vi "Handle Last Ack Core.vi"(4 "error in (no error)":errorcluster, 6 "Last Ack":refnum<class "Last Ack.lvclass">, 7 "Controller in":refnum<class "Controller.lvclass">) -> (0 "error out":errorcluster, 3 "Controller out":refnum<class "Controller.lvclass">)   [LabVIEW 2016, in "Controller Actor.lvlib" / "Controller.lvclass"]
doc: "(<B>Filename</B>: Actor Framework.lvlib:Actor.lvclass:Handle Last Ack Core.vi)\n\nDefines how the caller actor responds to the Last Ack message from a nested actor. The Last Ack message is the final message a nested actor sends to its caller before it shuts down. The message contains information about the final state of the nested actor.\n\nBy default, this method does nothing except return any error the nested actor sent. A descendant class may override this method to define behavior."
uses:
  <userlib>/Common Components/Controller/Controller.lvclass
  <vilib>/ActorFramework/LastAck/Last Ack.lvclass
  <vilib>/ActorFramework/LastAck/Last Ack.lvclass/Last Ack.ctl
  <userlib>/Configuration Dialog Actor/Configuration.lvclass
  <userlib>/Configuration Dialog Actor/Configuration.lvclass/Configuration.ctl
  <userlib>/Common Components/Controller/Controller.lvclass/Controller.ctl
  <vilib>/ActorFramework/Message Enqueuer/Message Enqueuer.lvclass/Message Enqueuer.ctl
  <userlib>/Common Components/Function Actor/Function.lvclass
  <userlib>/Common Components/Function Actor/Function.lvclass/Function.ctl
  <vilib>/ActorFramework/Message Enqueuer/Enqueue.vi
  <userlib>/Common Components/User Interface/Messages/Enable UI Msg/Enable UI Msg.lvclass
  C:/Program Files (x86)/National Instruments/LabVIEW 2016/vi.lib/ActorFramework/Message/Message.lvclass
  <vilib>/ActorFramework/Message Priority Queue/Priority Enqueue.vi
  <vilib>/ActorFramework/Actor/Actor.lvclass
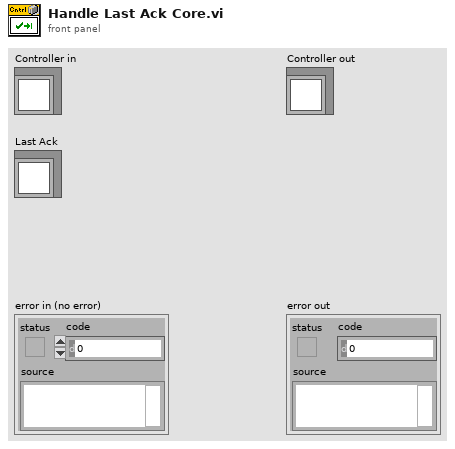
[diagram p1: front panel]
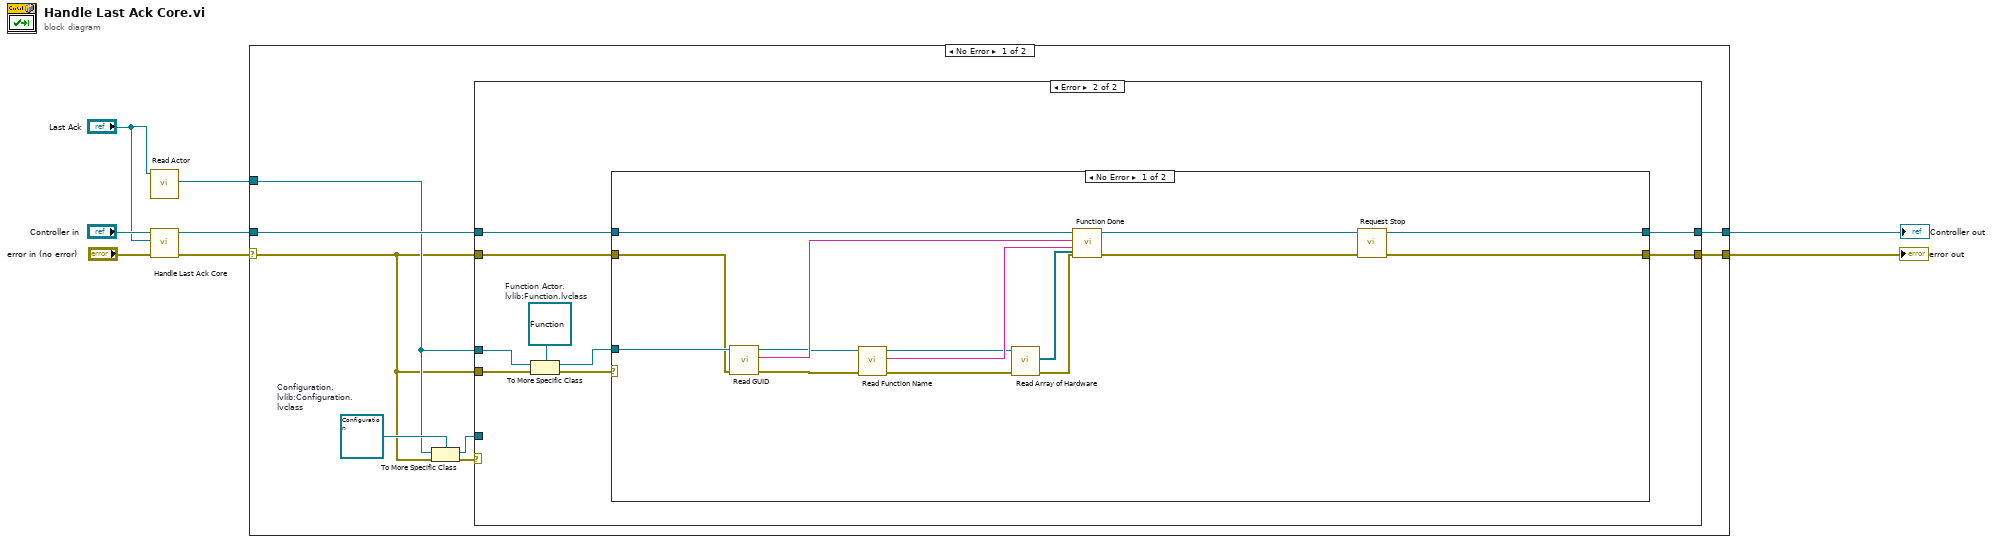
[diagram p0: block diagram]
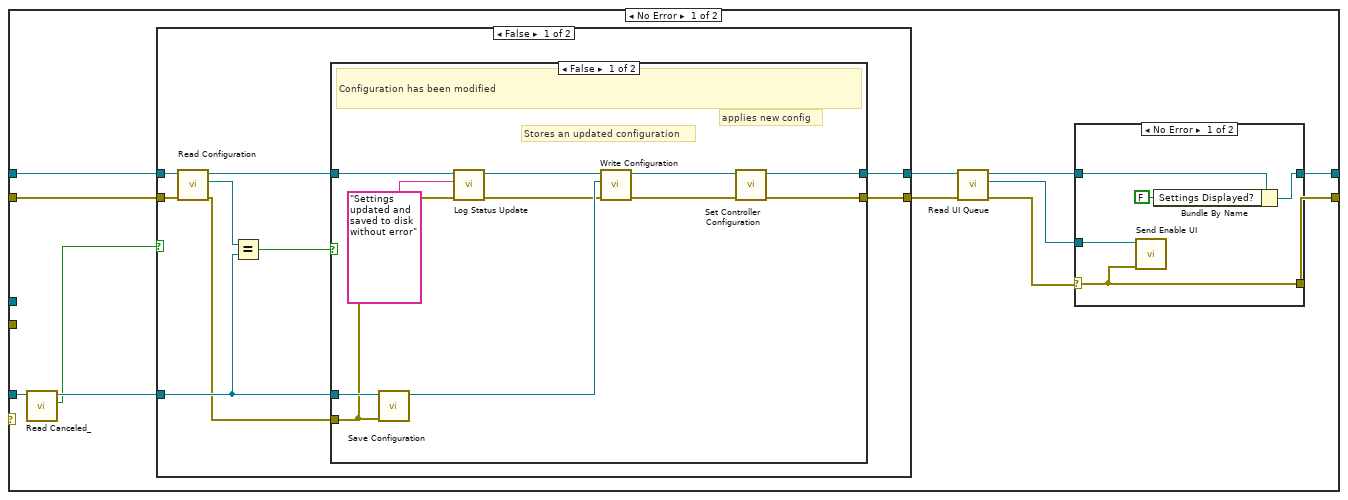
[diagram p2: hidden frame]
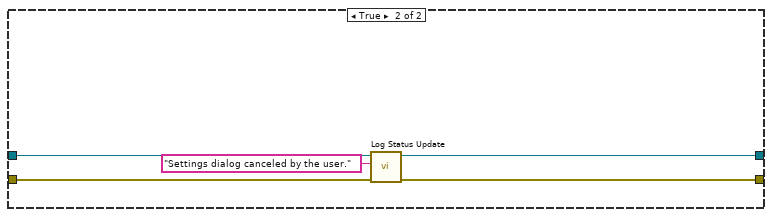
[diagram p4: hidden frame]
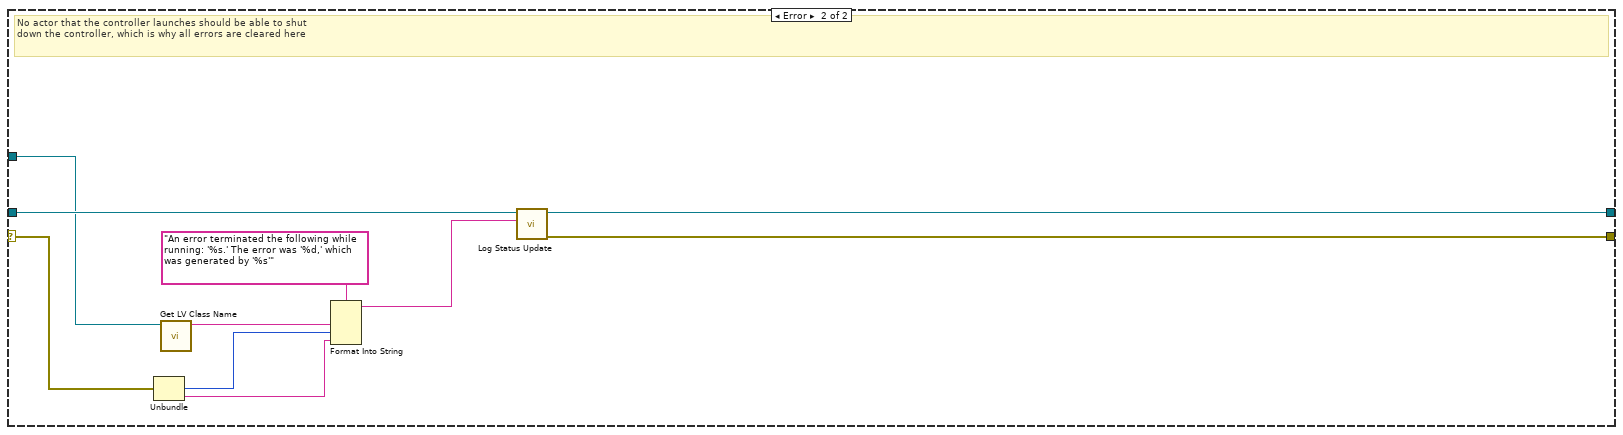
[diagram p7: hidden frame]
diagram:
  n1 = call <vilib>:"Read Actor.vi"("Last Ack"="Last Ack") -> ("Actor"=w3:refnum<class "Actor.lvclass">)  [unwired: 10 in]
  n2 = call-parent "Handle Last Ack Core.vi"("error in (no error)"="error in (no error)", "Last Ack"="Last Ack", "Actor in"="Controller in") -> ("error out"=w2:errorcluster, "Actor out"=w4:refnum<class "Controller.lvclass">)  [unwired: 3 in]
  n3 = case shown="No Error" w2 {
    selector: w2 -> [w9 w93]
    tunnel: [w16 w96] -> w7
    tunnel: [w15 w95] -> w5
    tunnel: w4 -> [w14 w97]
    tunnel: w3 -> [w10 w89]
    frame No Error {
      w11 = refnum<class "Configuration.lvclass"> refnum  # Configuration.lvlib:Configuration.lvclass
      n4 = To More Specific Class(target class=w11, reference=w10, error in=w9) -> (specific class reference=w13:refnum<class "Configuration.lvclass">, error out=w12:errorcluster)
      n5 = case shown="Error" w12 {
        tunnel: [w28 w63] -> w16
        tunnel: [w27 w62] -> w15
        tunnel: w14 -> [w26 w65]
        tunnel: w13 -> [w24 _]
        tunnel: w9 -> [w25 w64]
        tunnel: w10 -> [_ w70]
        tunnel: w9 -> [_ w69]
        frame No Error {
          n6 = call <vilib>:"Read Canceled_.vi"("Configuration in"=w24) -> ("Canceled?"=w17:bool, "Configuration out"=w23:refnum<class "Configuration.lvclass">)  [unwired: 8 in, 1 out]
          n7 = case shown="False" w17 {
            tunnel: w26 -> [w37 w52]
            tunnel: w25 -> [w36 w54]
            tunnel: w23 -> [w35 _]
            tunnel: [w30 w51] -> w19
            tunnel: [w29 w53] -> w18
            frame False {
              n8 = call <userlib>:"Read Configuration.vi"("error in (no error)"=w36, "Controller in"=w37) -> ("error out"=w34:errorcluster, "Configuration.lvlib:Configuration.lvclass"=w33:refnum<class "Configuration.lvclass">, "Controller out"=w31:refnum<class "Controller.lvclass">)  [unwired: 7 in]
              n9 = Equal?(x=w33, y=w35) -> (x = y?=w32:bool)
              n10 = case shown="False" w32 {
                tunnel: w35 -> [w47 _]
                tunnel: w34 -> [w44 w48]
                tunnel: w31 -> [w46 w49]
                tunnel: [w39 w49] -> w30
                tunnel: [w38 w48] -> w29
                frame False {
                  # "applies new config"
                  # "Stores an updated configuration"
                  # "Configuration has been modified"
                  n11 = call <userlib>:"Save Configuration.vi"("error in (no error)"=w44, "Configuration in"=w47) -> ("Configuration out"=w43:refnum<class "Configuration.lvclass">)  [unwired: 7 in, 2 out]
                  n12 = call-dynamic "Log Status Update.vi"("error in (no error)"=w44, "String"="Settings updated and saved to disk without error", "Controller in"=w46) -> ("error out"=w40:errorcluster, "Controller out"=w42:refnum<class "Controller.lvclass">)  [unwired: 7 in]
                  n13 = call <userlib>:"Write Configuration.vi"("Configuration.lvlib:Configuration.lvclass"=w43, "Controller in"=w42) -> ("Controller out"=w41:refnum<class "Controller.lvclass">)  [unwired: 8 in, 1 out]
                  n14 = call-dynamic "Set Controller Configuration.vi"("error in (no error)"=w40, "Controller in"=w41) -> ("error out"=w38:errorcluster, "Controller out"=w39:refnum<class "Controller.lvclass">)  [unwired: 8 in]
                }
                frame True {
                }
              }
            }
            frame True {
              n15 = call-dynamic "Log Status Update.vi"("error in (no error)"=w54, "String"="Settings dialog canceled by the user.", "Controller in"=w52) -> ("error out"=w53:errorcluster, "Controller out"=w51:refnum<class "Controller.lvclass">)  [unwired: 7 in]
            }
          }
          n16 = call <userlib>:"Read UI Queue.vi"("error in (no error)"=w18, "UI Controller in"=w19) -> ("error out"=w20:errorcluster, "UI Queue"=w22:refnum<class "Message Enqueuer.lvclass">, "UI Controller out"=w21:refnum<class "Controller.lvclass">)  [unwired: 7 in]
          n17 = case shown="No Error" w20 {
            selector: w20 -> [w55 w60]
            tunnel: w22 -> [w59 _]
            tunnel: w21 -> [w58 w61]
            tunnel: [w56 w61] -> w28
            tunnel: [w55 w60] -> w27
            frame No Error {
              n18 = call <userlib>:"Send Enable UI.vi"("error in (no error)"=w55, "Message Enqueuer"=w59) -> ()  [unwired: 8 in, 2 out]
              n19 = Bundle By Name(cluster=w58, "Settings Displayed?"=FALSE) -> (w56:refnum<class "Controller.lvclass">)
            }
            frame Error {
            }
          }
        }
        frame Error {
          w68 = refnum<class "Function.lvclass"> refnum  # Function Actor.lvlib:Function.lvclass
          n20 = To More Specific Class(target class=w68, reference=w70, error in=w69) -> (specific class reference=w66:refnum<class "Function.lvclass">, error out=w67:errorcluster)
          n21 = case shown="No Error" w67 {
            tunnel: w66 -> [w80 _]
            tunnel: w65 -> [w85 w87]
            tunnel: w64 -> [w76 w86]
            tunnel: [w71 w87] -> w63
            tunnel: [w73 w86] -> w62
            frame No Error {
              n22 = call <userlib>:"Read GUID.vi"("error in (no error)"=w76, "Function in"=w80) -> ("error out"=w75:errorcluster, "GUID"=w82:string, "Function out"=w79:refnum<class "Function.lvclass">)  [unwired: 7 in]
              n23 = call <userlib>:"Read Function Name.vi"("error in (no error)"=w75, "Function in"=w79) -> ("error out"=w74:errorcluster, "Function Name"=w81:string, "Function out"=w78:refnum<class "Function.lvclass">)  [unwired: 7 in]
              n24 = call <userlib>:"Read Array of Hardware.vi"("error in (no error)"=w74, "Function in"=w78) -> ("error out"=w77:errorcluster, "Array of Hardware"=w83:refnum<class "Hardware.lvclass">[])  [unwired: 7 in, 1 out]
              n25 = call-dynamic "Function Done.vi"("Array of Hardware"=w83, "error in (no error)"=w77, "Function Name"=w81, "GUID"=w82, "Controller in"=w85) -> ("error out"=w84:errorcluster, "Controller out"=w72:refnum<class "Controller.lvclass">)  [unwired: 5 in]
              n26 = call <userlib>:"Request Stop.vi"("error in (no error)"=w84, "Controller in"=w72) -> ("error out"=w73:errorcluster, "Controller out"=w71:refnum<class "Controller.lvclass">)  [unwired: 8 in]
            }
            frame Error {
            }
          }
        }
      }
    }
    frame Error {
      # "No actor that the controller launches should be able to shut\ndown the controller, which is why all errors are cleared here"
      n27 = Unbundle(w93) -> ("code"=w91:i32, "source"=w90:string)  [unwired: 1 out]
      n28 = call <vilib>:"Get LV Class Name.vi"("object"=w89) -> ("class name"=w88:string)  [unwired: 9 in, 1 out]
      n29 = Format Into String(format string="An error terminated the following while running: '%s.' The error was '%d,' which was generated by '%s'", w88, w91, w90) -> (resulting string=w94:string)  [unwired: 2 in, 1 out]
      n30 = call-dynamic "Log Status Update.vi"("String"=w94, "Controller in"=w97) -> ("error out"=w95:errorcluster, "Controller out"=w96:refnum<class "Controller.lvclass">)  [unwired: 8 in]
    }
  }
  "Controller out" <- w7
  "error out" <- w5
